vi "quack.vi"(8 "error in (no error)":errorcluster, 11 "Quack in":refnum<class "Quack.lvclass">) -> (0 "error out":errorcluster, 2 "String":string, 3 "Quack out":refnum<class "Quack.lvclass">)   [LabVIEW 2013, in "Quack.lvclass"]
uses:
  Quack.lvclass
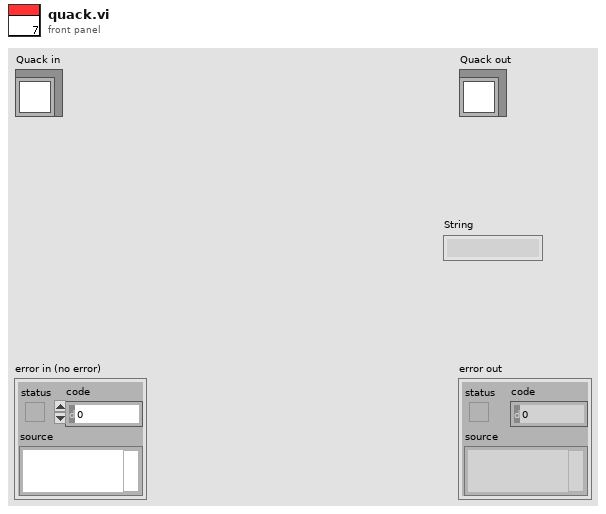
[diagram p1: front panel]
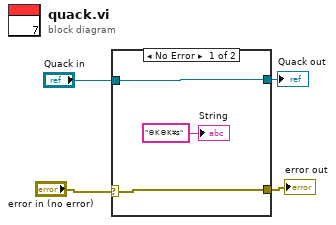
[diagram p0: block diagram]
diagram:
  n1 = case shown="No Error" "error in (no error)" {
    selector: "error in (no error)" -> [w6 w9]
    tunnel: [w6 w9] -> w3
    tunnel: [w5 w8] -> w2
    tunnel: "Quack in" -> [w5 w8]
    frame No Error {
      "String" <- "©K©K¥s" ("String")
    }
    frame Error {
    }
  }
  "error out" <- w3
  "Quack out" <- w2
